vi "2D Explorer.vi"() -> ()   [LabVIEW 2023]
doc: "Demonstrates how to find the extrema points (minima and maxima) and graph a two-variable equation."
uses:
  <vilib>/gmath/NI_Gmath.lvlib
panel:
  out "x":dbl format="%#.6g"
  out "y":dbl format="%#.6g"
  in  "option":u16(ring) items=["one minimum", "one maximum", "many minima", "many maxima"]
  in  "var":string[](array[string])=["x", "y"]
  out "Y":cluster{"Y Values":dbl[], "X2 Values":dbl[]}(graph)
  out "X":cluster{"X1 Values":dbl[], "Y Values":dbl[]}(graph)
  in  "Stop":bool
  out "Intensity Graph":dbl[][](graph)
  out "z":dbl format="%#.6g"
  out "value":dbl[](array[numeric]) format="%#_5g"
  out "optima":dbl[][](array[numeric])
  in  "end":dbl[](array[numeric])=[1.0, 1.0] format="%#.6g"
  in  "start":dbl[](array[numeric])=[0.0, 0.0] format="%#.6g"
  in  "formula":string="sin(3*x)*cos(5*y)"
  in  "# of points":u32=50
  # "Overview: Demonstrates the use of the Find All Minima nD VI to find the minimum or maximum values of a two dimensional function.\nRequirements: LabVIEW Full Development System\nInstructions:\n1. Run the VI.\n2. Observe the minimum and maximum values found.\n3. Click Stop to stop the VI."
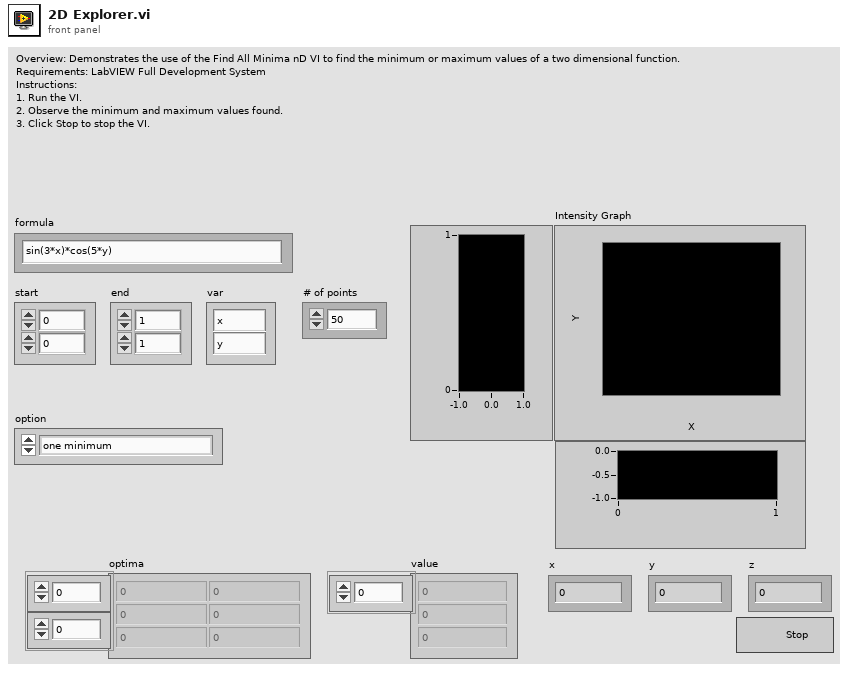
[diagram p1: front panel]
types:
  T1 = typedef "LVPointDoubleTypeDef.ctl" = cluster{"Cursor X":dbl, "Cursor Y":dbl}
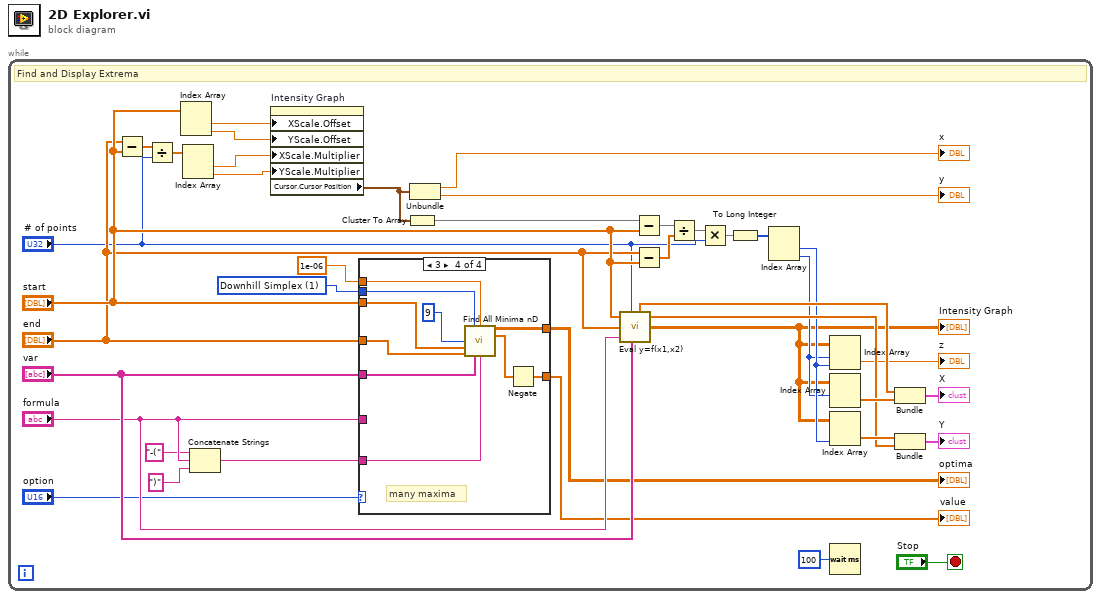
[diagram p0: block diagram]
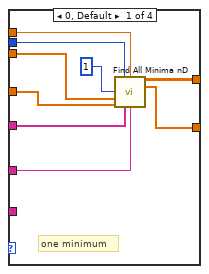
[diagram p2: hidden frame]
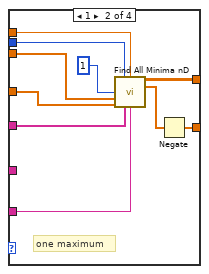
[diagram p3: hidden frame]
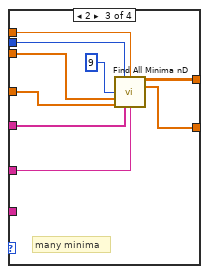
[diagram p4: hidden frame]
diagram:
  n1 = while {
    stop <- "Stop" stop-if-true
    w2 = u16 1 items=["Conjugate Gradient", "Downhill Simplex"] ("algorithm")
    # "Find and Display Extrema"
    n2 = Subtract(x="end", y="start") -> (x-y=w21:dbl[])
    n3 = Divide(x=w21, y="# of points") -> (x/y=w20:dbl[])
    n4 = Index Array(array="start") -> (element #1=w10:dbl, element #2=w9:dbl)  [unwired: 2 in]
    n5 = Index Array(array=w20) -> (element #1=w8:dbl, element #2=w7:dbl)  [unwired: 2 in]
    n6 = Concatenate Strings("-(", "formula", ")") -> (w31:string)
    n7 = property on="Intensity Graph" class="IntGraph (strict)"("XScale.Offset"=w10, "YScale.Offset"=w9, "XScale.Multiplier"=w8, "YScale.Multiplier"=w7) -> ("Cursor.Cursor Position"=w6:T1)  [unwired: 2 in, 2 out]
    n8 = case shown="3" "option" {
      tunnel: "start" -> [w44 w55 w65 w75]
      tunnel: "end" -> [w43 w54 w64 w74]
      tunnel: "var" -> [w48 w58 w68 w78]
      tunnel: [w46 w57 w67 w77] -> w30
      tunnel: [w49 w51 w61 w70] -> w34
      tunnel: w31 -> [_ w52 _ w71]
      tunnel: "formula" -> [w47 _ w62 _]
      tunnel: 1e-06 -> [w45 w56 w66 w76]
      tunnel: w2 -> [w42 w53 w63 w73]
      frame 0, Default {
        # "one minimum"
        n9 = call <vilib>:"Find All Minima nD.vi"("algorithm"=w42, "accuracy"=w45, "number of trials"=1, "Start"=w44, "End"=w43, "X"=w48, "F(X)"=w47) -> ("X Values"=w46:dbl[][], "F Values"=w49:dbl[])  [unwired: 5 in, 2 out]
      }
      frame 1 {
        # "one maximum"
        n10 = call <vilib>:"Find All Minima nD.vi"("algorithm"=w53, "accuracy"=w56, "number of trials"=1, "Start"=w55, "End"=w54, "X"=w58, "F(X)"=w52) -> ("X Values"=w57:dbl[][], "F Values"=w59:dbl[])  [unwired: 5 in, 2 out]
        n11 = Negate(x=w59) -> (-x=w51:dbl[])
      }
      frame 2 {
        # "many minima"
        n12 = call <vilib>:"Find All Minima nD.vi"("algorithm"=w63, "accuracy"=w66, "number of trials"=9, "Start"=w65, "End"=w64, "X"=w68, "F(X)"=w62) -> ("X Values"=w67:dbl[][], "F Values"=w61:dbl[])  [unwired: 5 in, 2 out]
      }
      frame 3 {
        # "many maxima"
        n13 = call <vilib>:"Find All Minima nD.vi"("algorithm"=w73, "accuracy"=w76, "number of trials"=9, "Start"=w75, "End"=w74, "X"=w78, "F(X)"=w71) -> ("X Values"=w77:dbl[][], "F Values"=w72:dbl[])  [unwired: 5 in, 2 out]
        n14 = Negate(x=w72) -> (-x=w70:dbl[])
      }
    }
    "optima" <- w30
    "value" <- w34
    n15 = Cluster To Array(cluster=w6) -> (array=w28:dbl[])
    n16 = Unbundle(w6) -> ("Cursor X"=→"x":dbl, "Cursor Y"=→"y":dbl)
    n17 = call <vilib>:"Eval y=f(x1,x2).vi"("Start"="start", "number of points"="# of points", "End"="end", "formula"="formula", "Variables"="var") -> ("X1 Values"=w18:dbl[], "X2 Values"=w17:dbl[], "Y Values"=w14:dbl[][])  [unwired: 2 out]
    "Intensity Graph" <- w14
    n18 = Subtract(x=w28, y="start") -> (x-y=w27:dbl[])
    n19 = Subtract(x="end", y="start") -> (x-y=w26:dbl[])
    n20 = Divide(x=w27, y=w26) -> (x/y=w25:dbl[])
    n21 = Multiply(x=w25, y="# of points") -> (x*y=w24:dbl[])
    n22 = To Long Integer(number=w24) -> (32bit integer=w23:i32[])
    n23 = Index Array(array=w23) -> (element #1=w16:i32, element #2=w15:i32)  [unwired: 2 in]
    n24 = Index Array(array=w14, index (row)=w15, index (col)=w16) -> (element=→"z":dbl)
    n25 = Index Array(array=w14, index (row)=w15) -> (element=w22:dbl[])  [unwired: 1 in]
    n26 = Index Array(array=w14, index (col)=w16) -> (element=w19:dbl[])  [unwired: 1 in]
    n27 = Wait (ms)(milliseconds to wait=u32 100) -> ()  [unwired: 1 out]
    n28 = Bundle("X1 Values"=w18, "Y Values"=w22) -> (→"X":cluster{"X1 Values":dbl[], "Y Values":dbl[]})  [unwired: 1 in]
    n29 = Bundle("Y Values"=w19, "X2 Values"=w17) -> (→"Y":cluster{"Y Values":dbl[], "X2 Values":dbl[]})  [unwired: 1 in]
  }
